vi "Do RSSI at 2.45 GHz.vi"(7 "Execute on Remote? (T)\nAKA on IMPLANT":bool=TRUE, 8 "error in":errorcluster, 9 "Gain Selection":T1(ring)=enum."Gain of 3", 10 "Number of RSSI Readings":i32=20, 11 "VISA Resource Name":refnum<visa-resource-name>) -> (0 "error out":errorcluster, 1 "min RSSI Value (2.45 GHz)":u8, 2 "mean RSSI Value (2.45 GHz)":dbl=nan format="%0.2f", 3 "dup VISA Resource Name":refnum<visa-resource-name>, 4 "max RSSI Value (2.45 GHz)":u8, 5 "2.45 GHz RSSI Values":u8[](array[numeric]))   [LabVIEW 2010]
uses:
  <vilib>/Analysis/NI_AALBase.lvlib
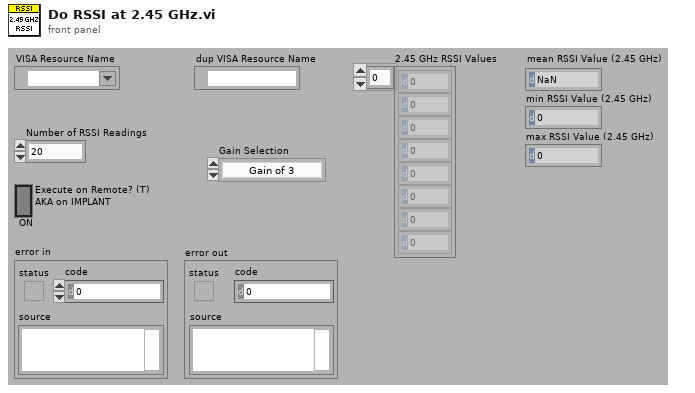
[diagram p1: front panel]
types:
  T1 = enum8{"Gain of 1", "Gain of 3", "Gain of 10", "Gain of 30"}
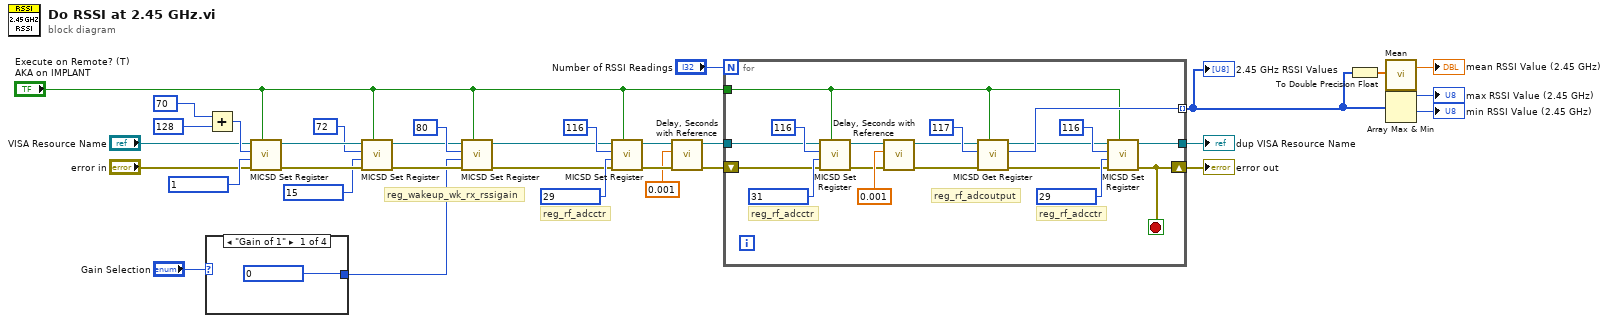
[diagram p0: block diagram]
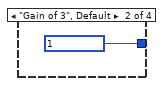
[diagram p2: hidden frame]
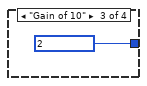
[diagram p3: hidden frame]
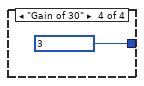
[diagram p4: hidden frame]
diagram:
  # "reg_rf_adcctr"
  # "reg_wakeup_wk_rx_rssigain"
  n1 = case shown="\"Gain of 1\"" "Gain Selection" {
    tunnel: [u8 0 ("Data") u8 1 ("Data") u8 2 ("Data") u8 3 ("Data")] -> w2
    frame "Gain of 1" {
    }
    frame "Gain of 3", Default {
    }
    frame "Gain of 10" {
    }
    frame "Gain of 30" {
    }
  }
  n2 = Add(x=u16 70, y=u16 128) -> (x+y=w31:u16)
  n3 = call "MICSD Set Register.vi"("Execute on Remote?(F)"="Execute on Remote? (T)\nAKA on IMPLANT", "error in (no error)"="error in", "Data"=u8 1, "Address"=w31, "VISA Resource Name"="VISA Resource Name") -> ("error out"=w30:errorcluster, "dup VISA Resource Name"=w29:refnum<visa-resource-name>)  [unwired: 5 in]
  n4 = call "MICSD Set Register.vi"("Execute on Remote?(F)"="Execute on Remote? (T)\nAKA on IMPLANT", "error in (no error)"=w30, "Data"=u8 15, "Address"=u16 72, "VISA Resource Name"=w29) -> ("error out"=w23:errorcluster, "dup VISA Resource Name"=w24:refnum<visa-resource-name>)  [unwired: 5 in]
  n5 = call "MICSD Set Register.vi"("Execute on Remote?(F)"="Execute on Remote? (T)\nAKA on IMPLANT", "error in (no error)"=w23, "Data"=w2, "Address"=u16 80, "VISA Resource Name"=w24) -> ("error out"=w19:errorcluster, "dup VISA Resource Name"=w20:refnum<visa-resource-name>)  [unwired: 5 in]
  n6 = call "MICSD Set Register.vi"("Execute on Remote?(F)"="Execute on Remote? (T)\nAKA on IMPLANT", "error in (no error)"=w19, "Data"=u8 29, "Address"=u16 116, "VISA Resource Name"=w20) -> ("error out"=w16:errorcluster, "dup VISA Resource Name"=w18:refnum<visa-resource-name>)  [unwired: 5 in]
  n7 = call "Delay, Seconds with Reference.vi"("error in"=w16, "delay"=dbl[unit] 0.001, "VISA resource"=w18) -> ("error out"=w15:errorcluster, "VISA resource dup"=w17:refnum<visa-resource-name>)  [unwired: 3 in, 1 out]
  n8 = for {
    N: "Number of RSSI Readings" -> [_]
    tunnel: w17 -> [w53]
    tunnel: [w45] -> w8 mode=indexing
    tunnel: [w40] -> w12
    shift-right: [w39] -> w11
    shift-left: w15 -> [w52]
    tunnel: "Execute on Remote? (T)\nAKA on IMPLANT" -> [w38]
    stop <- w39 stop-if-true
    # "reg_rf_adcctr"
    # "reg_rf_adcoutput"
    # "reg_rf_adcctr"
    n9 = call "MICSD Set Register.vi"("Execute on Remote?(F)"=w38, "error in (no error)"=w52, "Data"=u8 31, "Address"=u16 116, "VISA Resource Name"=w53) -> ("error out"=w49:errorcluster, "dup VISA Resource Name"=w50:refnum<visa-resource-name>)  [unwired: 5 in]
    n10 = call "Delay, Seconds with Reference.vi"("error in"=w49, "delay"=dbl[unit] 0.001, "VISA resource"=w50) -> ("error out"=w46:errorcluster, "VISA resource dup"=w47:refnum<visa-resource-name>)  [unwired: 3 in, 1 out]
    n11 = call "MICSD Get Register.vi"("Execute on Remote?(F)"=w38, "error in (no error)"=w46, "Address"=u16 117, "VISA Resource Name"=w47) -> ("error out"=w41:errorcluster, "Data"=w45:u8, "dup VISA Resource Name"=w42:refnum<visa-resource-name>)  [unwired: 5 in]
    n12 = call "MICSD Set Register.vi"("Execute on Remote?(F)"=w38, "error in (no error)"=w41, "Data"=u8 29, "Address"=u16 116, "VISA Resource Name"=w42) -> ("error out"=w39:errorcluster, "dup VISA Resource Name"=w40:refnum<visa-resource-name>)  [unwired: 5 in]
  }
  "2.45 GHz RSSI Values" <- w8
  "dup VISA Resource Name" <- w12
  "error out" <- w11
  n13 = To Double Precision Float(number=w8) -> (double precision float=w7:dbl[])
  n14 = call <vilib>:"Mean.vi"("X"=w7) -> ("mean"=→"mean RSSI Value (2.45 GHz)":dbl)  [unwired: 1 out]
  n15 = Array Max & Min(array=w8) -> (max value=→"max RSSI Value (2.45 GHz)":u8, min value=→"min RSSI Value (2.45 GHz)":u8)  [unwired: 2 out]
